vi "MReadRS232_2.vi"(0 "port1":i32, 1 "dev1":i32=1, 4 "port2":i32, 5 "dev2":i32=2, 7 "port3":i32, 8 "dev7":i32=5, 9 "dev8":i32, 10 "port7":i32, 11 "port8":i32, 12 "dev5":i32=5, 14 "port5":i32, 15 "dev4":i32=4, 16 "dev6":i32=5, 17 "port6":i32, 18 "port4":i32, 19 "dev3":i32=3) -> (6 "output array":dbl[](array[numeric]), 13 "params":dbl[](array[numeric]))   [LabVIEW 2016]
uses:
  BERTTA.dll
panel:
  # "MReadRS232(9, 1, 9, 2, 13, 3, 13, 4, 10, 5, 11, 5, 12, 5, 0, 0, res_vec);"
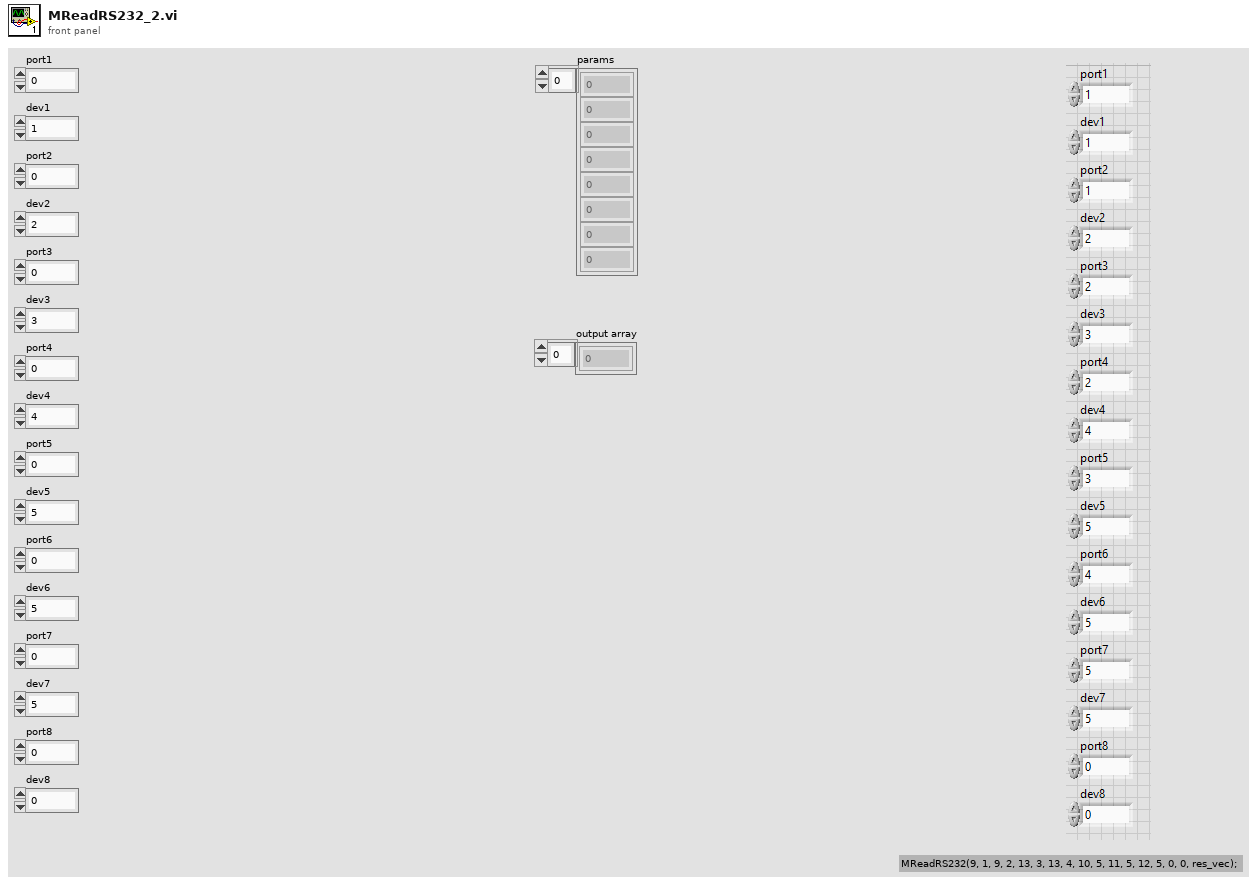
[diagram p1: front panel]
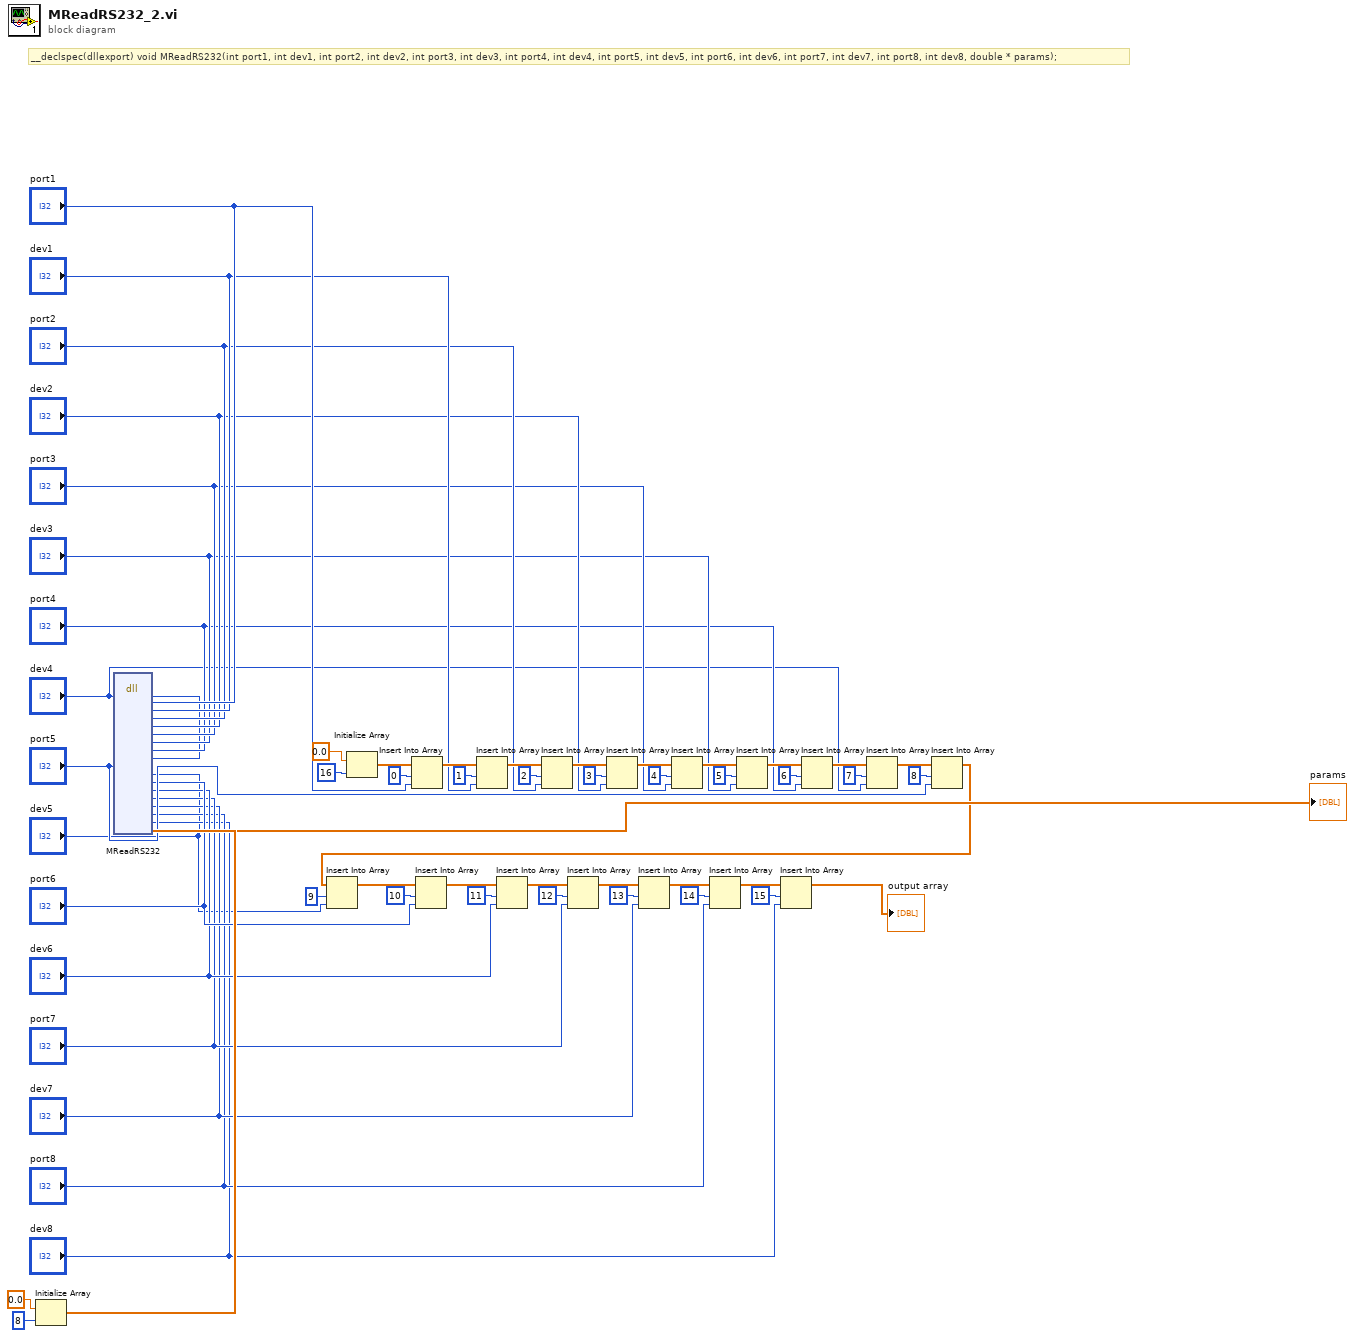
[diagram p0: block diagram]
diagram:
  # "__declspec(dllexport) void MReadRS232(int port1, int dev1, int port2, int dev2, int port3, int dev3, int port4, int dev4, int port5, int dev5, int port6, int dev6, int port7, int dev7, int port8, int dev8, double * params);"
  n1 = Initialize Array(0.0 ("element"), 8 ("dimension size")) -> (w55:dbl[])
  n2 = dll-call lib="C:/Users/shresplab/OneDrive - Kemira Oyj/Documents/GitHub/Bertta/BERTTA/x64/Debug/BERTTA.dll" fn="MReadRS232"("port1"="port1", "dev1"="dev1", "port2"="port2", "dev2"="dev2", "port3"="port3", "dev3"="dev3", "port4"="port4", "dev4"="dev4", "port5"="port5", "dev5"="dev5", "port6"="port6", "dev6"="dev6", "port7"="port7", "dev7"="dev7", "port8"="port8", "dev8"="dev8", "params"=w55) -> ("params"=→"params":dbl[])  [unwired: 20 in, 2 out]
  n3 = Initialize Array(0.0 ("element"), 16 ("dimension size")) -> (w49:dbl[])
  n4 = Insert Into Array(array=w49, index=0, new element="port1") -> (w45:dbl[])
  n5 = Insert Into Array(array=w45, index=1, new element="dev1") -> (w42:dbl[])
  n6 = Insert Into Array(array=w42, index=2, new element="port2") -> (w39:dbl[])
  n7 = Insert Into Array(array=w39, index=3, new element="dev2") -> (w36:dbl[])
  n8 = Insert Into Array(array=w36, index=4, new element="port3") -> (w33:dbl[])
  n9 = Insert Into Array(array=w33, index=5, new element="dev3") -> (w30:dbl[])
  n10 = Insert Into Array(array=w30, index=6, new element="port4") -> (w27:dbl[])
  n11 = Insert Into Array(array=w27, index=7, new element="dev4") -> (w24:dbl[])
  n12 = Insert Into Array(array=w24, index=8, new element="port5") -> (w4:dbl[])
  n13 = Insert Into Array(array=w4, index=9, new element="dev5") -> (w3:dbl[])
  n14 = Insert Into Array(array=w3, index=10, new element="port6") -> (w7:dbl[])
  n15 = Insert Into Array(array=w7, index=11, new element="dev6") -> (w17:dbl[])
  n16 = Insert Into Array(array=w17, index=12, new element="port7") -> (w14:dbl[])
  n17 = Insert Into Array(array=w14, index=13, new element="dev7") -> (w11:dbl[])
  n18 = Insert Into Array(array=w11, index=14, new element="port8") -> (w8:dbl[])
  n19 = Insert Into Array(array=w8, index=15, new element="dev8") -> (→"output array":dbl[])
